vi "Execution Engine.vi"(7 "Hierarchy":string, 10 "Event Queue":refnum<queue>, 11 "Reg Event Queue":refnum<queue>) -> ()   [LabVIEW 2022 SP3, in "FlexBlocks Support.lvlib"]
uses:
  FlexBlocks Support.lvlib
  Execution Events.ctl
  Worker Registration.ctl
  Worker Block.ctl
  Block Status with Error.ctl
  Block Status.ctl
  Block State.ctl
  Block Phase.ctl
  Block Command.ctl
  <extravilib>/ChannelInstances/Messenger-t'FlexBlocks Support.lvlib-Execution Events.ctl'/Write With Abort.vi
  <extravilib>/ChannelInstances/Messenger-t'FlexBlocks Support.lvlib-Execution Events.ctl'/Endpoint.vi
panel:
  out "Status":T2(array[cluster])
  in  "Close":bool
  in  "Stop":bool
  in  "Step":bool
  in  "Run":bool
  in  "Init":bool
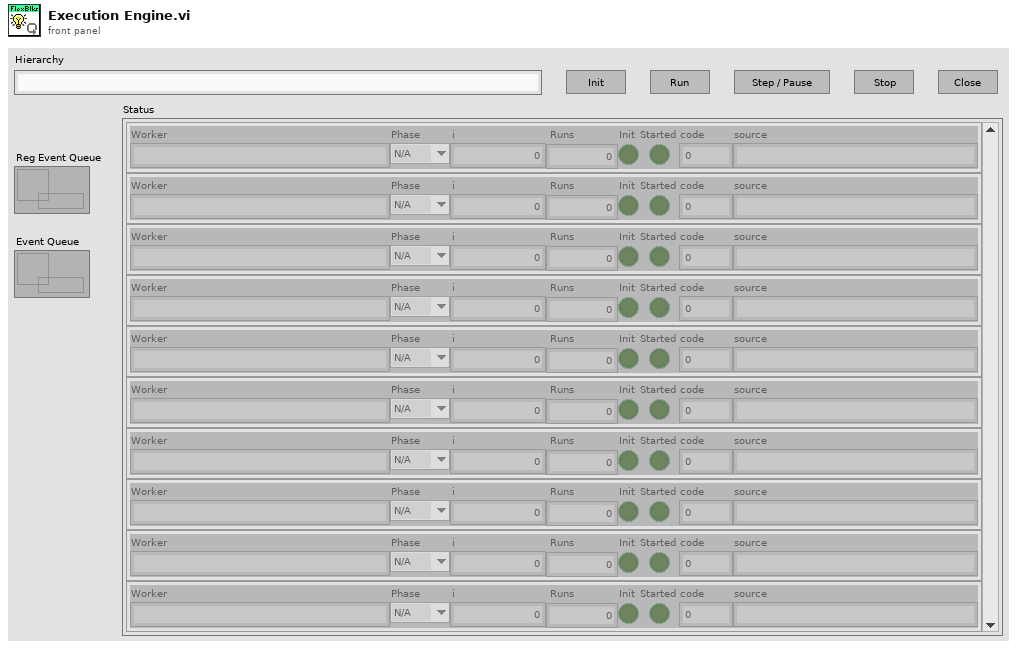
[diagram p1: front panel]
types:
  T1 = typedef "FlexBlocks Support.lvlib/Block Phase.ctl" = enum16{"N/A", "Read", "Work", "Write"}
  T2 = cluster{"Worker":string, "Phase":T1, "i":i32, "Runs":u32, "Init":bool, "Started":bool, "code":i32, "source":string}[]
  T3 = typedef "FlexBlocks Support.lvlib/Worker Block.ctl" = cluster{"Block Status":refnum<user-event>, "Command Queue":refnum<queue>, "Status":T4}
  T4 = typedef "FlexBlocks Support.lvlib/Block Status with Error.ctl" = cluster{"Block Status":T5, "Error":errorcluster}
  T5 = typedef "FlexBlocks Support.lvlib/Block Status.ctl" = cluster{"State":T6, "Next State":T6, "Runs":u32, "i":i32, "Init":bool, "Started":bool, "Closing":bool, "Step":bool, "Phase":T1, "Worker":string}
  T6 = typedef "FlexBlocks Support.lvlib/Block State.ctl" = enum16{"Idle", "Init", "Start", "Run", "Stop", "Close"}
  T7 = typedef "FlexBlocks Support.lvlib/Execution Events.ctl" = cluster{"Registration":refnum<user-event>, "Init":refnum<user-event>, "Run":refnum<user-event>, "Step":refnum<user-event>, "Stop":refnum<user-event>, "Close":refnum<user-event>, "Block Status":refnum<user-event>}
  T8 = typedef "FlexBlocks Support.lvlib/Block Command.ctl" = enum16{"Close", "Init", "Step", "Run", "Pause"}
  T9 = cluster{"Worker":string, "Phase":T1, "i":i32, "Runs":u32, "Init":bool, "Started":bool, "code":i32, "source":string}
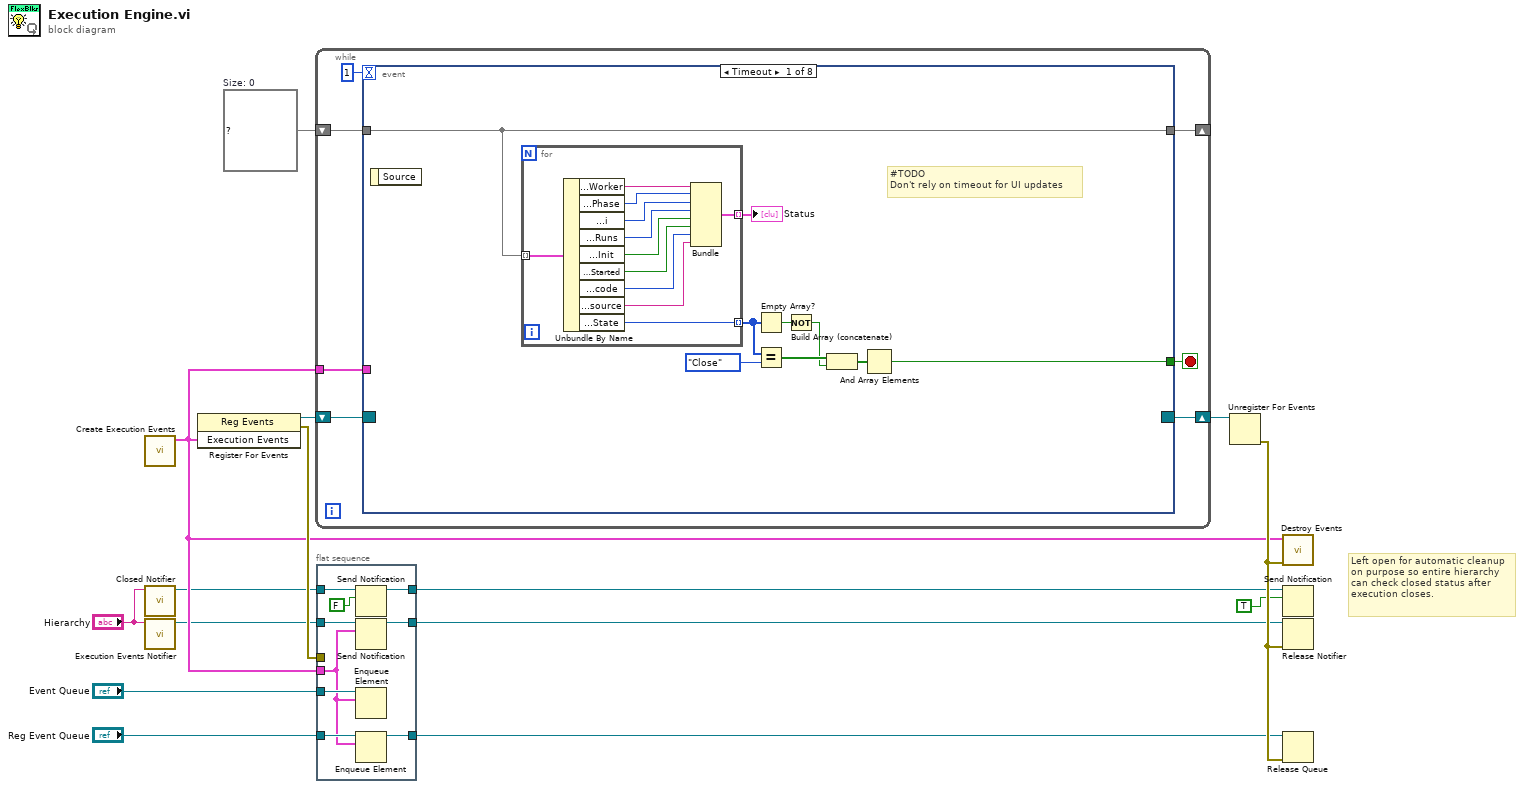
[diagram p0: block diagram]
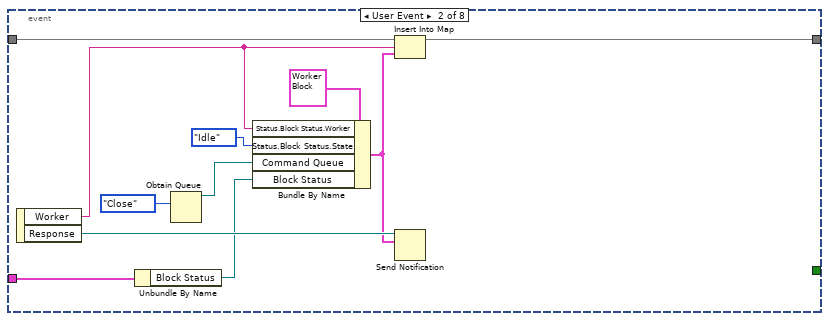
[diagram p2: hidden frame]
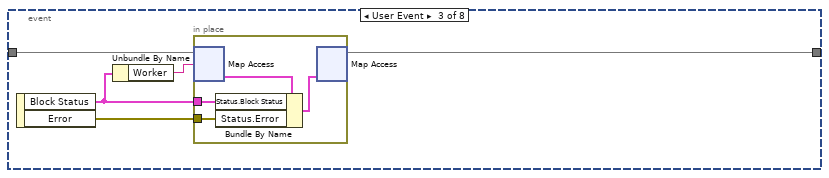
[diagram p3: hidden frame]
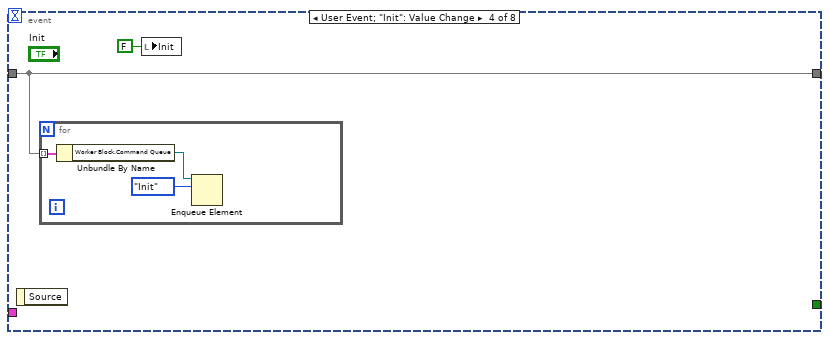
[diagram p4: hidden frame]
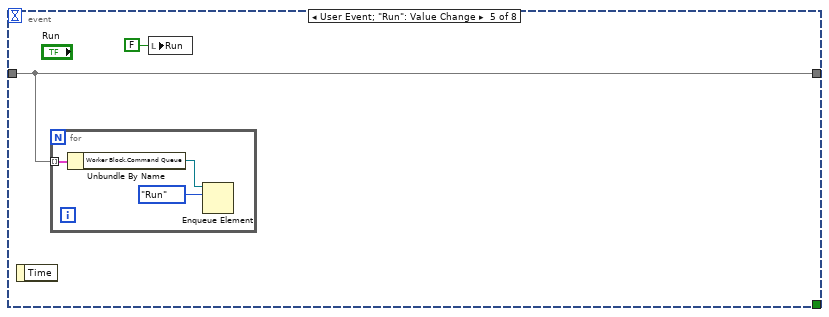
[diagram p5: hidden frame]
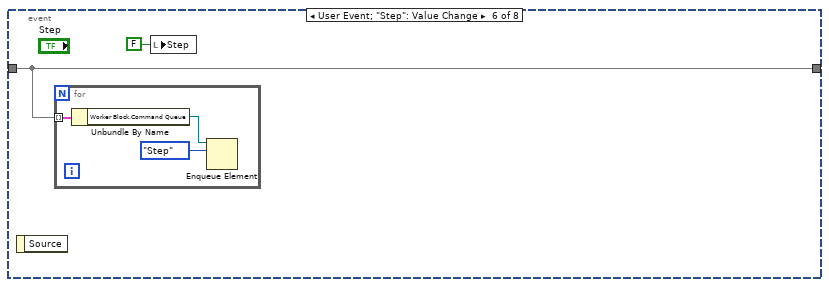
[diagram p6: hidden frame]
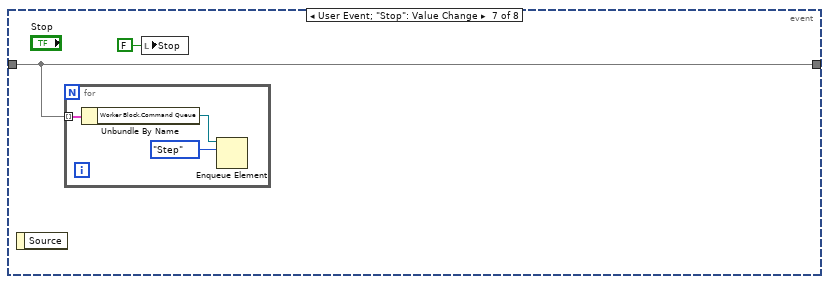
[diagram p7: hidden frame]
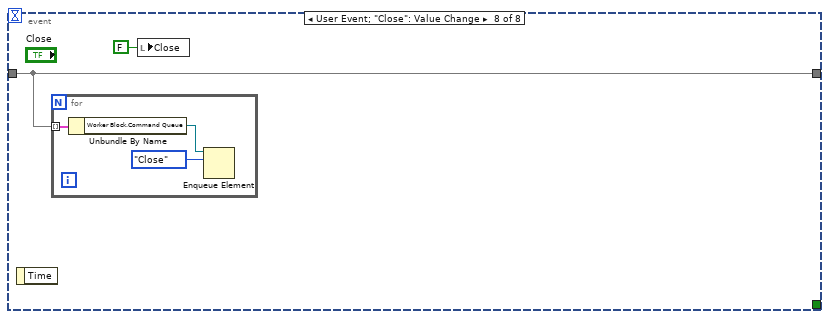
[diagram p8: hidden frame]
diagram:
  w11 = map{string, T3} {}  # Size: 0
  # "Left open for automatic cleanup on purpose so entire hierarchy can check closed status after execution closes."
  n1 = call "Create Execution Events.vi"() -> ("Execution Events"=w8:T7)  [unwired: 11 in]
  n2 = call "Closed Notifier.vi"("Hierarchy (Auto)"="Hierarchy") -> ("Closed Notifier"=w5:refnum<notifier>)  [unwired: 10 in]
  n3 = call "Execution Events Notifier.vi"("Hierarchy (Auto)"="Hierarchy") -> ("Events Notifier"=w7:refnum<notifier>)  [unwired: 9 in, 1 out]
  n4 = register-events(w8) -> (reference out=w12:refnum<event-registration>, error out=w14:errorcluster)  [unwired: 2 in]
  n5 = while {
    shift-right: [w20] -> w10
    shift-left: w12 -> [w21]
    shift-right: [w17] -> _
    shift-left: w11 -> [w18]
    tunnel: w8 -> [w16]
    stop <- w19 stop-if-true
    n6 = event shown="[0] Timeout" {
      selector: w21 -> [_ _ _ _ _ _ _ _]
      dyn-events: [_ _ _ _ _ _ _ _] -> w20
      timeout: 1 -> [_ _ _ _ _ _ _ _]
      tunnel: [w27 _ _ _ _ _ _ _] -> w19
      tunnel: w18 -> [w31 w49 w58 w64 w68 w73 w78 w83]
      tunnel: [w31 w47 w54 w64 w68 w73 w78 w83] -> w17
      tunnel: w16 -> [_ w44 _ _ _ _ _ _]
      event Timeout {
        # "#TODO\nDon't rely on timeout for UI updates"
        n7 = event-data() -> ()  [unwired: 1 in, 1 out]
        n8 = for {
          tunnel: w31 -> [w42] mode=indexing
          tunnel: [w33] -> w30 mode=indexing
          tunnel: [w32] -> w26 mode=indexing
          n9 = Unbundle By Name(w42) -> ("Worker Block.Status.Block Status.Worker"=w41:string, "Worker Block.Status.Block Status.Phase"=w40:T1, "Worker Block.Status.Block Status.i"=w39:i32, "Worker Block.Status.Block Status.Runs"=w38:u32, "Worker Block.Status.Block Status.Init"=w37:bool, "Worker Block.Status.Block Status.Started"=w36:bool, "Worker Block.Status.Error.code"=w35:i32, "Worker Block.Status.Error.source"=w34:string, "Worker Block.Status.Block Status.State"=w32:T6)
          n10 = Bundle("Worker"=w41, "Phase"=w40, "i"=w39, "Runs"=w38, "Init"=w37, "Started"=w36, "code"=w35, "source"=w34) -> (w33:T9)  [unwired: 1 in]
        }
        "Status" <- w30
        n11 = Empty Array?(array=w26) -> (empty?=w25:bool)
        n12 = Equal?(x=w26, y=Block_State."Close" ("Worker Block.Status.Block Status.State")) -> (x = y?=w28:bool[])
        n13 = Not(x=w25) -> (.not. x?=w23:bool)
        n14 = Build Array (concatenate)(w28, w23) -> (w24:bool[])
        n15 = And Array Elements(Boolean array=w24) -> (logical AND=w27:bool)
      }
      event User Event {
        n16 = event-data() -> ("Worker"=w46:string, "Response"=w48:refnum<notifier>)  [unwired: 1 in]
        n17 = Unbundle By Name(w44) -> ("Block Status"=w43:refnum<user-event>)
        n18 = Obtain Queue(element data type=Block_Command."Close" ("Block Command")) -> (queue out=w51:refnum<queue>)  [unwired: 4 in, 2 out]
        n19 = Bundle By Name(cluster=T3 {"Block Status"=refnum, "Command Queue"=refnum, "Status"={"Block Status"={"State"=enum."Idle", "Next State"=enum."Idle", "Runs"=0, "i"=0, "Init"=FALSE, "Started"=FALSE, "Closing"=FALSE, "Step"=FALSE, "Phase"=enum."N/A", "Worker"=""}, "Error"={"status"=FALSE, "code"=0, "source"=""}}} ("Worker Block"), "Status.Block Status.Worker"=w46, "Status.Block Status.State"=Block_State."Idle" ("Block Status with Error.Block Status.State"), "Command Queue"=w51, "Block Status"=w43) -> (w45:T3)
        n20 = Insert Into Map(map in=w49, key=w46, value=w45) -> (map out=w47:map{string, T3})  [unwired: 2 out]
        n21 = Send Notification(notification=w45, notifier=w48) -> ()  [unwired: 1 in, 2 out]
      }
      event User Event {
        n22 = event-data() -> ("Block Status"=w56:T5, "Error"=w55:errorcluster)  [unwired: 1 in]
        n23 = Unbundle By Name(w56) -> ("Worker"=w57:string)
        n24 = in-place {
          in-place-border: w56 -> [w61]
          in-place-border: w55 -> [w60]
          n25 = in-place-map #1(w58, w57) -> (w62:T3)  [unwired: 1 in, 1 out]
          n26 = Bundle By Name(cluster=w62, "Status.Block Status"=w61, "Status.Error"=w60) -> (w59:T3)
          n27 = in-place-map #1(w59) -> (w54:map{string, T3})  [unwired: 1 in, 2 out]
        }
      }
      event User Event; "Init": Value Change {
        n28 = event-data() -> ()  [unwired: 1 in, 1 out]
        n29 = for {
          tunnel: w64 -> [w67] mode=indexing
          n30 = Unbundle By Name(w67) -> ("Worker Block.Command Queue"=w66:refnum<queue>)
          n31 = Enqueue Element(queue=w66, element=Block_Command."Init") -> ()  [unwired: 2 in, 3 out]
        }
        n32 = local write "Init"(FALSE ("Init")) -> ()
      }
      event User Event; "Run": Value Change {
        n33 = event-data() -> ()  [unwired: 1 in, 1 out]
        n34 = for {
          tunnel: w68 -> [w72] mode=indexing
          n35 = Unbundle By Name(w72) -> ("Worker Block.Command Queue"=w71:refnum<queue>)
          n36 = Enqueue Element(queue=w71, element=Block_Command."Run") -> ()  [unwired: 2 in, 3 out]
        }
        n37 = local write "Run"(FALSE ("Run")) -> ()
      }
      event User Event; "Step": Value Change {
        n38 = event-data() -> ()  [unwired: 1 in, 1 out]
        n39 = for {
          tunnel: w73 -> [w77] mode=indexing
          n40 = Unbundle By Name(w77) -> ("Worker Block.Command Queue"=w76:refnum<queue>)
          n41 = Enqueue Element(queue=w76, element=Block_Command."Step") -> ()  [unwired: 2 in, 3 out]
        }
        n42 = local write "Step"(FALSE ("Step")) -> ()
      }
      event User Event; "Stop": Value Change {
        n43 = event-data() -> ()  [unwired: 1 in, 1 out]
        n44 = for {
          tunnel: w78 -> [w82] mode=indexing
          n45 = Unbundle By Name(w82) -> ("Worker Block.Command Queue"=w81:refnum<queue>)
          n46 = Enqueue Element(queue=w81, element=Block_Command."Step") -> ()  [unwired: 2 in, 3 out]
        }
        n47 = local write "Stop"(FALSE ("Stop")) -> ()
      }
      event User Event; "Close": Value Change {
        n48 = event-data() -> ()  [unwired: 1 in, 1 out]
        n49 = for {
          tunnel: w83 -> [w87] mode=indexing
          n50 = Unbundle By Name(w87) -> ("Worker Block.Command Queue"=w86:refnum<queue>)
          n51 = Enqueue Element(queue=w86, element=Block_Command."Close") -> ()  [unwired: 2 in, 3 out]
        }
        n52 = local write "Close"(FALSE ("Close")) -> ()
      }
    }
  }
  n53 = flat-sequence {
    tunnel: w14 -> [_]
    tunnel: w8 -> [w88]
    tunnel: "Reg Event Queue" -> [w96]
    tunnel: [w95] -> w9
    tunnel: w7 -> [w94]
    tunnel: [w93] -> w6
    tunnel: w5 -> [w92]
    tunnel: [w90] -> w3
    tunnel: "Event Queue" -> [w89]
    frame #0 {
      n54 = Send Notification(notification=FALSE, notifier=w92) -> (notifier out=w90:refnum<notifier>)  [unwired: 1 in, 1 out]
      n55 = Send Notification(notification=w88, notifier=w94) -> (notifier out=w93:refnum<notifier>)  [unwired: 1 in, 1 out]
      n56 = Enqueue Element(queue=w89, element=w88) -> ()  [unwired: 2 in, 3 out]
      n57 = Enqueue Element(queue=w96, element=w88) -> (queue out=w95:refnum<queue>)  [unwired: 2 in, 2 out]
    }
  }
  n58 = Unregister For Events(event registration refnum=w10) -> (error out=w15:errorcluster)  [unwired: 1 in]
  n59 = call "Destroy Events.vi"("error in (no error)"=w15, "Execution Events"=w8) -> ()  [unwired: 10 in]
  n60 = Send Notification(notification=TRUE, notifier=w3) -> ()  [unwired: 1 in, 2 out]
  n61 = Release Notifier(notifier=w6, error in (no error)=w15) -> ()  [unwired: 1 in, 3 out]
  n62 = Release Queue(queue=w9, error in (no error)=w15) -> ()  [unwired: 1 in, 3 out]
